vi "Example.vi"() -> ()   [LabVIEW 2013, in "TS.lvlib"]
doc: "Non-reentrant."
uses:
  TS.lvlib
panel:
  out "Found 2":bool
  out "Value Out 2":dbl
  out "Value Out":dbl
  out "Found":bool
  in  "Value":dbl
  out "Error Out":errorcluster
  in  "Error In":errorcluster
  in  "Name":string="My - DBL"
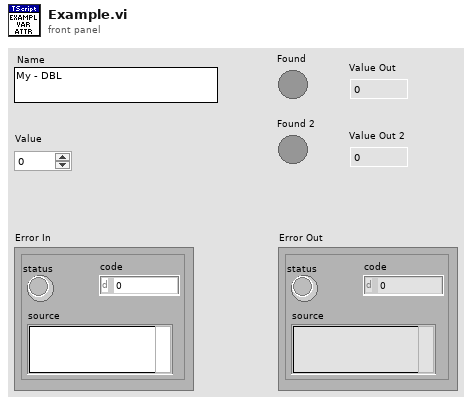
[diagram p1: front panel]
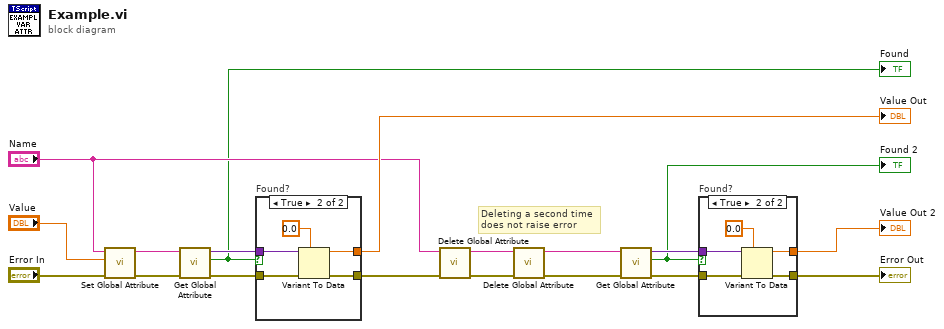
[diagram p0: block diagram]
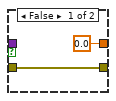
[diagram p2: hidden frame]
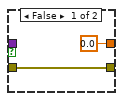
[diagram p3: hidden frame]
diagram:
  # "Deleting a second time\ndoes not raise error"
  n1 = call "Set Global Attribute.vi"("Error In"="Error In", "Value"="Value", "Name"="Name") -> ("Error Out"=w18:errorcluster, "dup Name"=w17:string)  [unwired: 7 in]
  n2 = call "Get Global Attribute.vi"("Error In"=w18, "Name"=w17) -> ("Error Out"=w13:errorcluster, "Found"=w6:bool, "Value"=w15:variant)  [unwired: 7 in]
  "Found" <- w6
  n3 = case "Found?" shown="True" w6 {
    tunnel: w15 -> [_ w26]
    tunnel: [0.0 w24] -> w14
    tunnel: w13 -> [w21 w23]
    tunnel: [w21 w22] -> w12
    frame False {
    }
    frame True {
      n4 = Variant To Data(error in=w23, type=0.0, Variant=w26) -> (data=w24:dbl, error out=w22:errorcluster)
    }
  }
  "Value Out" <- w14
  n5 = call "Delete Global Attribute.vi"("Error In"=w12, "Name"="Name") -> ("Error Out"=w2:errorcluster, "dup Name"=w4:string)  [unwired: 8 in]
  n6 = call "Delete Global Attribute.vi"("Error In"=w2, "Name"=w4) -> ("Error Out"=w1:errorcluster, "dup Name"=w3:string)  [unwired: 8 in]
  n7 = call "Get Global Attribute.vi"("Error In"=w1, "Name"=w3) -> ("Error Out"=w10:errorcluster, "Found"=w5:bool, "Value"=w9:variant)  [unwired: 7 in]
  "Found 2" <- w5
  n8 = case "Found?" shown="True" w5 {
    tunnel: w10 -> [w27 w33]
    tunnel: w9 -> [_ w31]
    tunnel: [w27 w30] -> w8
    tunnel: [0.0 w29] -> w7
    frame False {
    }
    frame True {
      n9 = Variant To Data(error in=w33, type=0.0, Variant=w31) -> (data=w29:dbl, error out=w30:errorcluster)
    }
  }
  "Error Out" <- w8
  "Value Out 2" <- w7
